vi "q3 half adder.vi"(8 "B":bool, 11 "A":bool) -> (0 "CARRY":bool, 3 "SUM":bool)   [LabVIEW 2025]
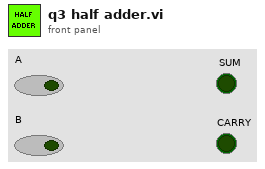
[diagram p1: front panel]
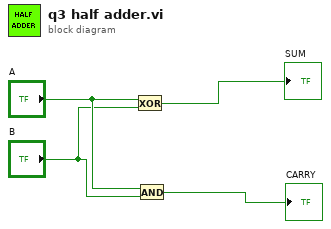
[diagram p0: block diagram]
diagram:
  n1 = Exclusive Or(1:"B", 2:"A") -> (0:→"SUM":bool)
  n2 = And(x="A", y="B") -> (x .and. y?=→"CARRY":bool)
